vi "Columns.vi"() -> (2 "Definition":T1)   [LabVIEW 2020, in "Conditum-Example.lvlib" / "User.lvclass"]
uses:
  User.lvclass
  Conditum/Columns/String/String.lvclass
  Conditum/Columns/Integer/Integer.lvclass
  Conditum/Columns/Timestamp/Timestamp.lvclass
  Conditum/Columns/Boolean/Boolean.lvclass
  Conditum/Columns/Entity Collection/Entity Collection.lvclass
  Conditum/Columns/String/String Definition.ctl
  Conditum/Columns/Type/Definition.ctl
  Conditum/Attributes.ctl
  Conditum/Columns/String/Definition.ctl
  Conditum/Columns/Integer/Integer Definition.ctl
  Conditum/Columns/Integer/Definition.ctl
  Conditum/Columns/Timestamp/Timestamp Definition.ctl
  Conditum/Columns/Timestamp/Definition.ctl
  Conditum/Columns/Boolean/Boolean Definition.ctl
  Conditum/Columns/Boolean/Definition.ctl
  Conditum/Columns/Entity Collection/Collection Definition.ctl
  Conditum/Columns/Relation/Relation Info.ctl
  Conditum/Relation Mapping.ctl
  Game/Game.lvclass
  User.lvclass/User.ctl
  Conditum/Conditum.lvlib
  Conditum/Columns/Type/Type.lvclass
  Conditum/Entity/Entity.lvclass
  Conditum/Columns/Relation/Definition.ctl
  Conditum/Columns/Relation/Relation.lvclass
  Conditum/Columns/Relation/Entity Relation Definition.ctl
  C:/dev/lv20CE/lv-conditum/Conditum/Entity/Entity.lvclass
  C:/dev/lv20CE/lv-conditum/Conditum-Example/Game/Game.lvclass
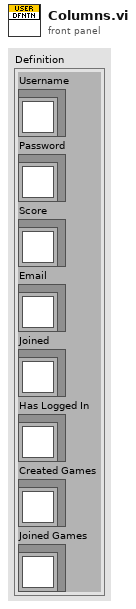
[diagram p1: front panel]
types:
  T1 = cluster{"Username":refnum<class "String.lvclass">, "Password":refnum<class "String.lvclass">, "Score":refnum<class "Integer.lvclass">, "Email":refnum<class "String.lvclass">, "Joined":refnum<class "Timestamp.lvclass">, "Has Logged In":refnum<class "Boolean.lvclass">, "Created Games":refnum<class "Entity Collection.lvclass">, "Joined Games":refnum<class "Entity Collection.lvclass">}
  T2 = typedef "Conditum.lvlib/Columns.lvlib/Relation.lvclass/Entity Relation Definition.ctl" = cluster{"Type":T3, "Entity":T4}
  T3 = typedef "Conditum.lvlib/Columns.lvlib/Type.lvclass/Definition.ctl" = cluster{"Name":string, "Nullable":bool, "Default NULL":bool}
  T4 = typedef "Conditum.lvlib/Columns.lvlib/Relation.lvclass/Definition.ctl" = cluster{"Reversed By":string, "Mapping":T5, "Entity":refnum<class "Entity.lvclass">}
  T5 = typedef "Conditum.lvlib/Relation Mapping.ctl" = enum16{"OneToMany", "ManyToOne", "ManyToMany", "OneToOne"}
  T6 = typedef "Conditum.lvlib/Columns.lvlib/Entity Collection.lvclass/Collection Definition.ctl" = cluster{"Table Name":string, "Relation":T7}
  T7 = typedef "Conditum.lvlib/Relation Info.ctl" = cluster{"Mapping":T5, "Related To":string, "Reversed By":string}
  T8 = typedef "Conditum.lvlib/Columns.lvlib/Boolean.lvclass/Boolean Definition.ctl" = cluster{"Type":T3, "Attributes":T9, "Boolean":T10}
  T9 = typedef "Conditum.lvlib/Attributes.ctl" = cluster{"Primary Key":bool, "Unique":bool, "Foreign Key":bool, "Auto Increment":bool}
  T10 = typedef "Conditum.lvlib/Columns.lvlib/Boolean.lvclass/Definition.ctl" = cluster{"Default":bool}
  T11 = typedef "Conditum.lvlib/Columns.lvlib/Timestamp.lvclass/Timestamp Definition.ctl" = cluster{"Type":T3, "Attributes":T9, "Timestamp":T12}
  T12 = typedef "Conditum.lvlib/Columns.lvlib/Timestamp.lvclass/Definition.ctl" = cluster{"Default":timestamp}
  T13 = typedef "Conditum.lvlib/Columns.lvlib/String.lvclass/String Definition.ctl" = cluster{"Type":T3, "Attributes":T9, "String":T14}
  T14 = typedef "Conditum.lvlib/Columns.lvlib/String.lvclass/Definition.ctl" = cluster{"Default":string, "Length":i32}
  T15 = typedef "Conditum.lvlib/Columns.lvlib/Integer.lvclass/Integer Definition.ctl" = cluster{"Type":T3, "Attributes":T9, "Integer":T16}
  T16 = typedef "Conditum.lvlib/Columns.lvlib/Integer.lvclass/Definition.ctl" = cluster{"Default":i64}
  T17 = cluster{"String out":refnum<class "String.lvclass">, "String out":refnum<class "String.lvclass">, "Integer out":refnum<class "Integer.lvclass">, "String out":refnum<class "String.lvclass">, "DateTime out":refnum<class "Timestamp.lvclass">, "Boolean out":refnum<class "Boolean.lvclass">, "Entity Collection out":refnum<class "Entity Collection.lvclass">, "Entity Collection out":refnum<class "Entity Collection.lvclass">}
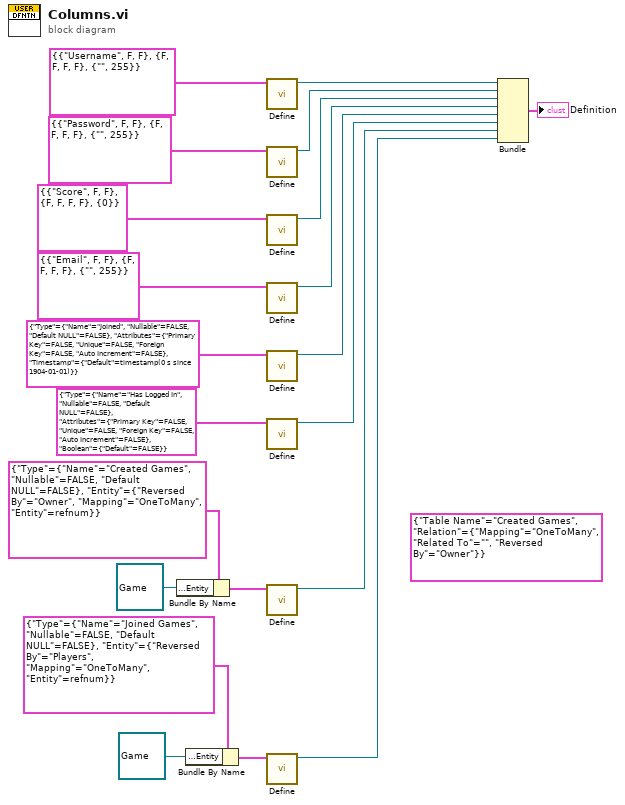
[diagram p0: block diagram]
diagram:
  (unwired) T6 {"Table Name"="Created Games", "Relation"={"Mapping"=enum."OneToMany", "Related To"="", "Reversed By"="Owner"}} ("Collection Definition")
  n1 = Bundle By Name(cluster=T2 {"Type"={"Name"="Created Games", "Nullable"=FALSE, "Default NULL"=FALSE}, "Entity"={"Reversed By"="Owner", "Mapping"=enum."OneToMany", "Entity"=refnum}} ("Entity Relation Definition"), "Entity.Entity"=refnum<class "Game.lvclass"> refnum ("Conditum-Example.lvlib:Game.lvclass")) -> (w2:T2)
  n2 = Bundle By Name(cluster=T2 {"Type"={"Name"="Joined Games", "Nullable"=FALSE, "Default NULL"=FALSE}, "Entity"={"Reversed By"="Players", "Mapping"=enum."OneToMany", "Entity"=refnum}} ("Entity Relation Definition"), "Entity.Entity"=refnum<class "Game.lvclass"> refnum ("Conditum-Example.lvlib:Game.lvclass")) -> (w4:T2)
  n3 = call "Define.vi"("Definition"=T13 {"Type"={"Name"="Username", "Nullable"=FALSE, "Default NULL"=FALSE}, "Attributes"={"Primary Key"=FALSE, "Unique"=FALSE, "Foreign Key"=FALSE, "Auto Increment"=FALSE}, "String"={"Default"="", "Length"=255}}) -> ("String out"=w15:refnum<class "String.lvclass">)  [unwired: 10 in]
  n4 = call "Define.vi"("Definition"=T13 {"Type"={"Name"="Password", "Nullable"=FALSE, "Default NULL"=FALSE}, "Attributes"={"Primary Key"=FALSE, "Unique"=FALSE, "Foreign Key"=FALSE, "Auto Increment"=FALSE}, "String"={"Default"="", "Length"=255}}) -> ("String out"=w14:refnum<class "String.lvclass">)  [unwired: 10 in]
  n5 = call "Define.vi"("Integer Definition"=T15 {"Type"={"Name"="Score", "Nullable"=FALSE, "Default NULL"=FALSE}, "Attributes"={"Primary Key"=FALSE, "Unique"=FALSE, "Foreign Key"=FALSE, "Auto Increment"=FALSE}, "Integer"={"Default"=0}}) -> ("Integer out"=w13:refnum<class "Integer.lvclass">)  [unwired: 10 in]
  n6 = call "Define.vi"("Definition"=T13 {"Type"={"Name"="Email", "Nullable"=FALSE, "Default NULL"=FALSE}, "Attributes"={"Primary Key"=FALSE, "Unique"=FALSE, "Foreign Key"=FALSE, "Auto Increment"=FALSE}, "String"={"Default"="", "Length"=255}}) -> ("String out"=w12:refnum<class "String.lvclass">)  [unwired: 10 in]
  n7 = call "Define.vi"("Definition"=T11 {"Type"={"Name"="Joined", "Nullable"=FALSE, "Default NULL"=FALSE}, "Attributes"={"Primary Key"=FALSE, "Unique"=FALSE, "Foreign Key"=FALSE, "Auto Increment"=FALSE}, "Timestamp"={"Default"=timestamp(0 s since 1904-01-01)}}) -> ("DateTime out"=w11:refnum<class "Timestamp.lvclass">)  [unwired: 10 in]
  n8 = call "Define.vi"("Init Data"=T8 {"Type"={"Name"="Has Logged In", "Nullable"=FALSE, "Default NULL"=FALSE}, "Attributes"={"Primary Key"=FALSE, "Unique"=FALSE, "Foreign Key"=FALSE, "Auto Increment"=FALSE}, "Boolean"={"Default"=FALSE}}) -> ("Boolean out"=w10:refnum<class "Boolean.lvclass">)  [unwired: 10 in]
  n9 = call "Define.vi"("Entity Relation Definition"=w2) -> ("Entity Collection out"=w9:refnum<class "Entity Collection.lvclass">)  [unwired: 10 in]
  n10 = call "Define.vi"("Entity Relation Definition"=w4) -> ("Entity Collection out"=w8:refnum<class "Entity Collection.lvclass">)  [unwired: 10 in]
  n11 = Bundle("String out"=w15, "String out"=w14, "Integer out"=w13, "String out"=w12, "DateTime out"=w11, "Boolean out"=w10, "Entity Collection out"=w9, "Entity Collection out"=w8) -> (→"Definition":T17)  [unwired: 1 in]
